vi "publish -- pll parameters.vi"(7 "publisher action":T3, 11 "pll parameters":T1={"PID mode"=enum."normal", "plot hist time (sec)"=1.0, "dt (sec)"=0.001, "visc hist time (sec)"=2.0, "time int ave time (sec)"=0.3, "PLL limits (Hz)"=5000.0} {"PLL limits (Hz)" format="%#.2f"; "time int ave time (sec)" format="%#_10f"; "visc hist time (sec)" format="%#_10f"; "dt (sec)" format="%#_10f"; "plot hist time (sec)" format="%#_10f"}) -> (3 "pll parameters OUT":T1={"PID mode"=enum."normal", "plot hist time (sec)"=1.0, "dt (sec)"=0.001, "visc hist time (sec)"=2.0, "time int ave time (sec)"=0.3, "PLL limits (Hz)"=5000.0} {"PLL limits (Hz)" format="%#.2f"; "time int ave time (sec)" format="%#_10f"; "visc hist time (sec)" format="%#_10f"; "dt (sec)" format="%#_10f"; "plot hist time (sec)" format="%#_10f"})   [LabVIEW 2018]
uses:
  PID - mode.ctl
  pll parameters.ctl
  publisher action.ctl
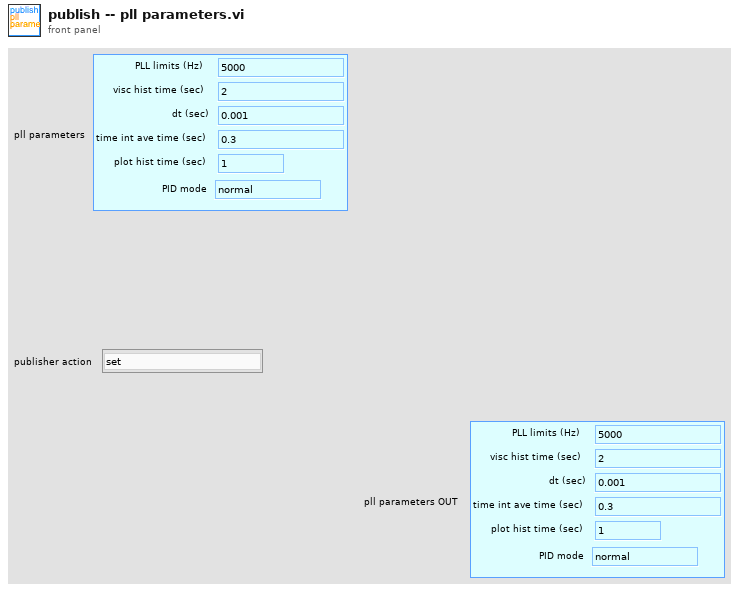
[diagram p1: front panel]
types:
  T1 = typedef "pll parameters.ctl" = cluster{"PID mode":T2, "plot hist time (sec)":dbl, "dt (sec)":dbl, "visc hist time (sec)":dbl, "time int ave time (sec)":dbl, "PLL limits (Hz)":dbl}
  T2 = typedef "PID - mode.ctl" = enum16{"normal", "heat"}
  T3 = typedef "publisher action.ctl" = enum16{"set", "get", "init", "check"}
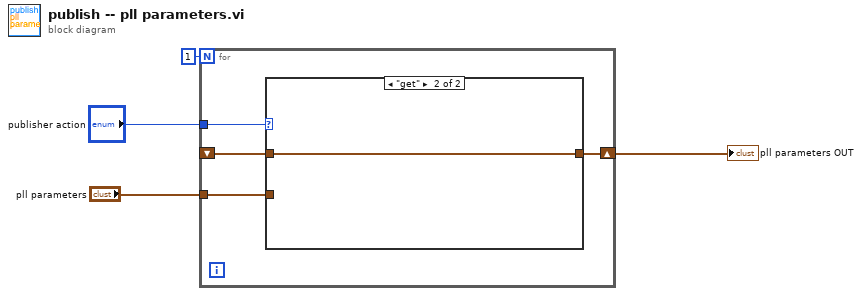
[diagram p0: block diagram]
diagram:
  n1 = for {
    N: 1 -> [_]
    tunnel: "publisher action" -> [w8]
    tunnel: "pll parameters" -> [w6]
    shift-right: [w7] -> w1
    shift-left: _ -> [w5]
    n2 = case shown="\"get\"" w8 {
      tunnel: [w9 w10] -> w7
      tunnel: w6 -> [w9 _]
      tunnel: w5 -> [_ w10]
      frame "set", Default {
      }
      frame "get" {
      }
    }
  }
  "pll parameters OUT" <- w1
